vi "Do.vi"(8 "error in":errorcluster, 10 "Actor in":refnum<class "Actor.lvclass">, 11 "Change Frequency MSG":refnum<class "Change Frequency MSG.lvclass">) -> (0 "error out":errorcluster, 2 "Actor out":refnum<class "Actor.lvclass">)   [LabVIEW 2014, in "Calibration.lvlib" / "Change Frequency MSG.lvclass"]
doc: "(<B>Filename</B>: Actor Framework.lvlib:Message.lvclass:Do.vi)\n\nDefines what a message does when it is received by an actor. Generally, a message instructs an actor to invoke one of its methods. By default, this method does nothing. A child class must override it to define behavior. Create a child class by using the Actor Framework Message Maker dialog box."
uses:
  Change Frequency MSG.lvclass
  <vilib>/ActorFramework/Actor/Actor.lvclass
  Change Frequency MSG.lvclass/Change Frequency MSG.ctl
  O3 Frequency Train Actor.lvclass
  SuperActor/Ex Nested.lvclass/Ex Nested.ctl
  O3 Frequency Train Actor.lvclass/O3 Frequency Train Actor.ctl
  SuperActor/Read Log Session.vi
  Accessors/Read FreqNotifier.vi
  <userlib>/_Session Fwk/Session - Root.lvclass
  reusable/Session APIs/Session Log/System Log.lvclass
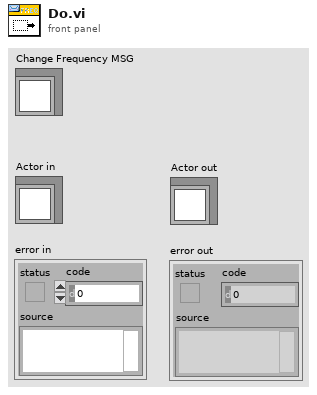
[diagram p1: front panel]
types:
  T1 = typedef "Session - Root.lvclass/Session Handle.ctl" = refnum<data-value>
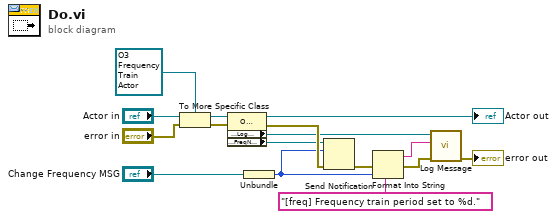
[diagram p0: block diagram]
diagram:
  n1 = To More Specific Class(target class=refnum<class "O3 Frequency Train Actor.lvclass"> refnum ("Calibration.lvlib:O3 Frequency Train Actors"), reference="Actor in", error in="error in") -> (specific class reference=w13:refnum<class "O3 Frequency Train Actor.lvclass">, error out=w12:errorcluster)
  n2 = property class="O3 Frequency Train Actors"(reference=w13, error in=w12) -> (reference out=→"Actor out":refnum<class "O3 Frequency Train Actor.lvclass">, error out=w10:errorcluster, "Accessors:Log Session"=w4:T1, "Accessors:FreqNotifier"=w5:refnum<notifier>)
  n3 = Unbundle("Change Frequency MSG") -> (w2:i64)
  n4 = Send Notification(notification=w2, notifier=w5, error in (no error)=w10) -> (error out=w1:errorcluster)  [unwired: 1 out]
  n5 = Format Into String(format string="[freq] Frequency train period set to %d.", error in=w1, w2) -> (resulting string=w7:string, error out=w8:errorcluster)  [unwired: 1 in]
  n6 = call "Log Message.vi"("error in"=w8, "MSG In"=w7, "session in"=w4) -> ("error out"=→"error out":errorcluster)  [unwired: 7 in, 1 out]
